vi "Parse GSV Params.vi"(11 "Fields In":string[](array[string])) -> (0 "Total SVs":i32, 1 "Message Num":i32, 2 "Total Messages":i32, 3 "Fields":string[](array[string]))   [LabVIEW 2020, in "nmea.lvlib" / "nmea.lvclass"]
uses:
  nmea.lvclass
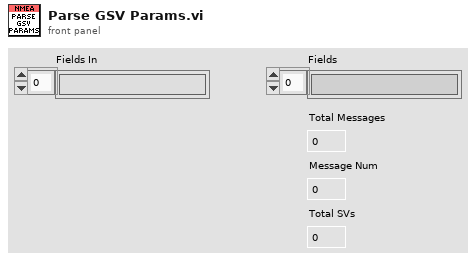
[diagram p1: front panel]
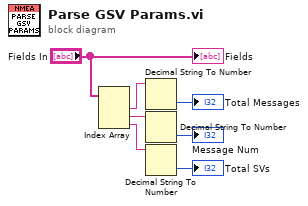
[diagram p0: block diagram]
diagram:
  n1 = Index Array(array="Fields In") -> (element #1=w6:string, element #2=w5:string, element #3=w4:string)  [unwired: 3 in]
  n2 = Decimal String To Number(string=w6) -> (number=→"Total Messages":i32)  [unwired: 2 in, 1 out]
  n3 = Decimal String To Number(string=w5) -> (number=→"Message Num":i32)  [unwired: 2 in, 1 out]
  n4 = Decimal String To Number(string=w4) -> (number=→"Total SVs":i32)  [unwired: 2 in, 1 out]
  "Fields" <- "Fields In"
